vi "Set CD Engine Event Ref.vi"(10 "CD Engine Event Ref":T1, 11 "Assembler in":refnum<class "Assembler.lvclass">) -> (3 "Assembler out":refnum<class "Assembler.lvclass">)   [LabVIEW 2019, in "TimingDRV Engine.lvlib" / "Assembler.lvclass"]
uses:
  Assembler.lvclass
  <vilib>/NI VeriStand/Custom Device API/Custom Device Engine Event Ref.ctl
  Assembler.lvclass/Assembler.ctl
  <vilib>/NI VeriStand/Custom Device API/Custom Device API.lvlib
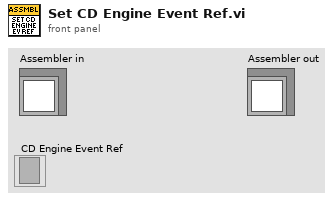
[diagram p1: front panel]
types:
  T1 = typedef "Custom Device API.lvlib/Custom Device Engine Event Ref.ctl" = refnum<event-registration>
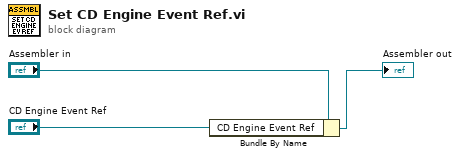
[diagram p0: block diagram]
diagram:
  n1 = Bundle By Name(cluster="Assembler in", "CD Engine Event Ref"="CD Engine Event Ref") -> (→"Assembler out":refnum<class "Assembler.lvclass">)
